vi "String Array to Spreadsheet Item.vi"(11 "Strings [] (ASCII)":string[](array[string])) -> (2 "Spreadsheet Item (ASCII)":string)   [LabVIEW 2013, in "SET Project Data.lvlib"]
uses:
  SET Project Data.lvlib
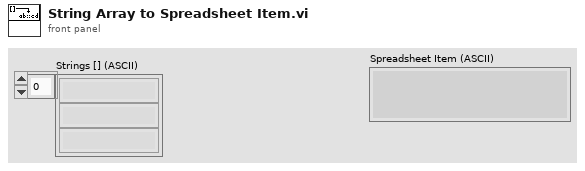
[diagram p1: front panel]
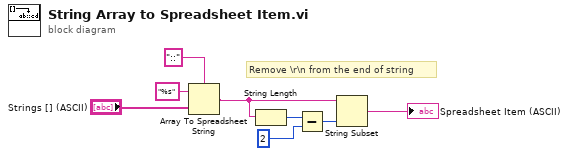
[diagram p0: block diagram]
diagram:
  # "Remove \\r\\n from the end of string"
  n1 = Array To Spreadsheet String(delimiter (Tab)="::", array="Strings [] (ASCII)", 3:"%s" ("format string")) -> (spreadsheet string=w3:string)
  n2 = String Length(string=w3) -> (length=w5:i32)
  n3 = Subtract(x=w5, y=2) -> (x-y=w6:i32)
  n4 = String Subset(string=w3, length (rest)=w6) -> (substring=→"Spreadsheet Item (ASCII)":string)  [unwired: 1 in]
